vi "Autonomous Independent.vi"() -> ()   [LabVIEW 2020]
doc: "This VI is called when autonomous begins, and will automatically be terminated when autonomous ends. You can carry out timed or sensor driven robot movement independently without needing to return to the caller."
uses:
  <vilib>/Rock Robotics/WPI/ThirdParty/REV Robotics/REVLib/Typedef/Spark MAX Control Type.ctl
  <vilib>/Rock Robotics/WPI/Utilities/WPI_GetSetVariantRefNum.vi
  <vilib>/Rock Robotics/Network Tables/NT Read String.vi
  <vilib>/Rock Robotics/Network Tables/NT Write Numeric Array.vi
panel:
  in  "Array of robot movements 2":T1(array[cluster])=[{"X Joystick Value"=0.39393939393939403, "Y Joystick Value"=0.0, "Delay (sec)"=1.0, "Movement Name"="turn"}, {"X Joystick Value"=-0.3737373737373737, "Y Joystick Value"=0.0, "Delay (sec)"=1.0, "Movement Name"="turn back"}] {"Y Joystick Value" scale=1.0..-1.0; "X Joystick Value" scale=-1.0..1.0}
  # "Be sure to right-click and choose Data Operations>>Make Current Value default if you want to save the array values with the VI"
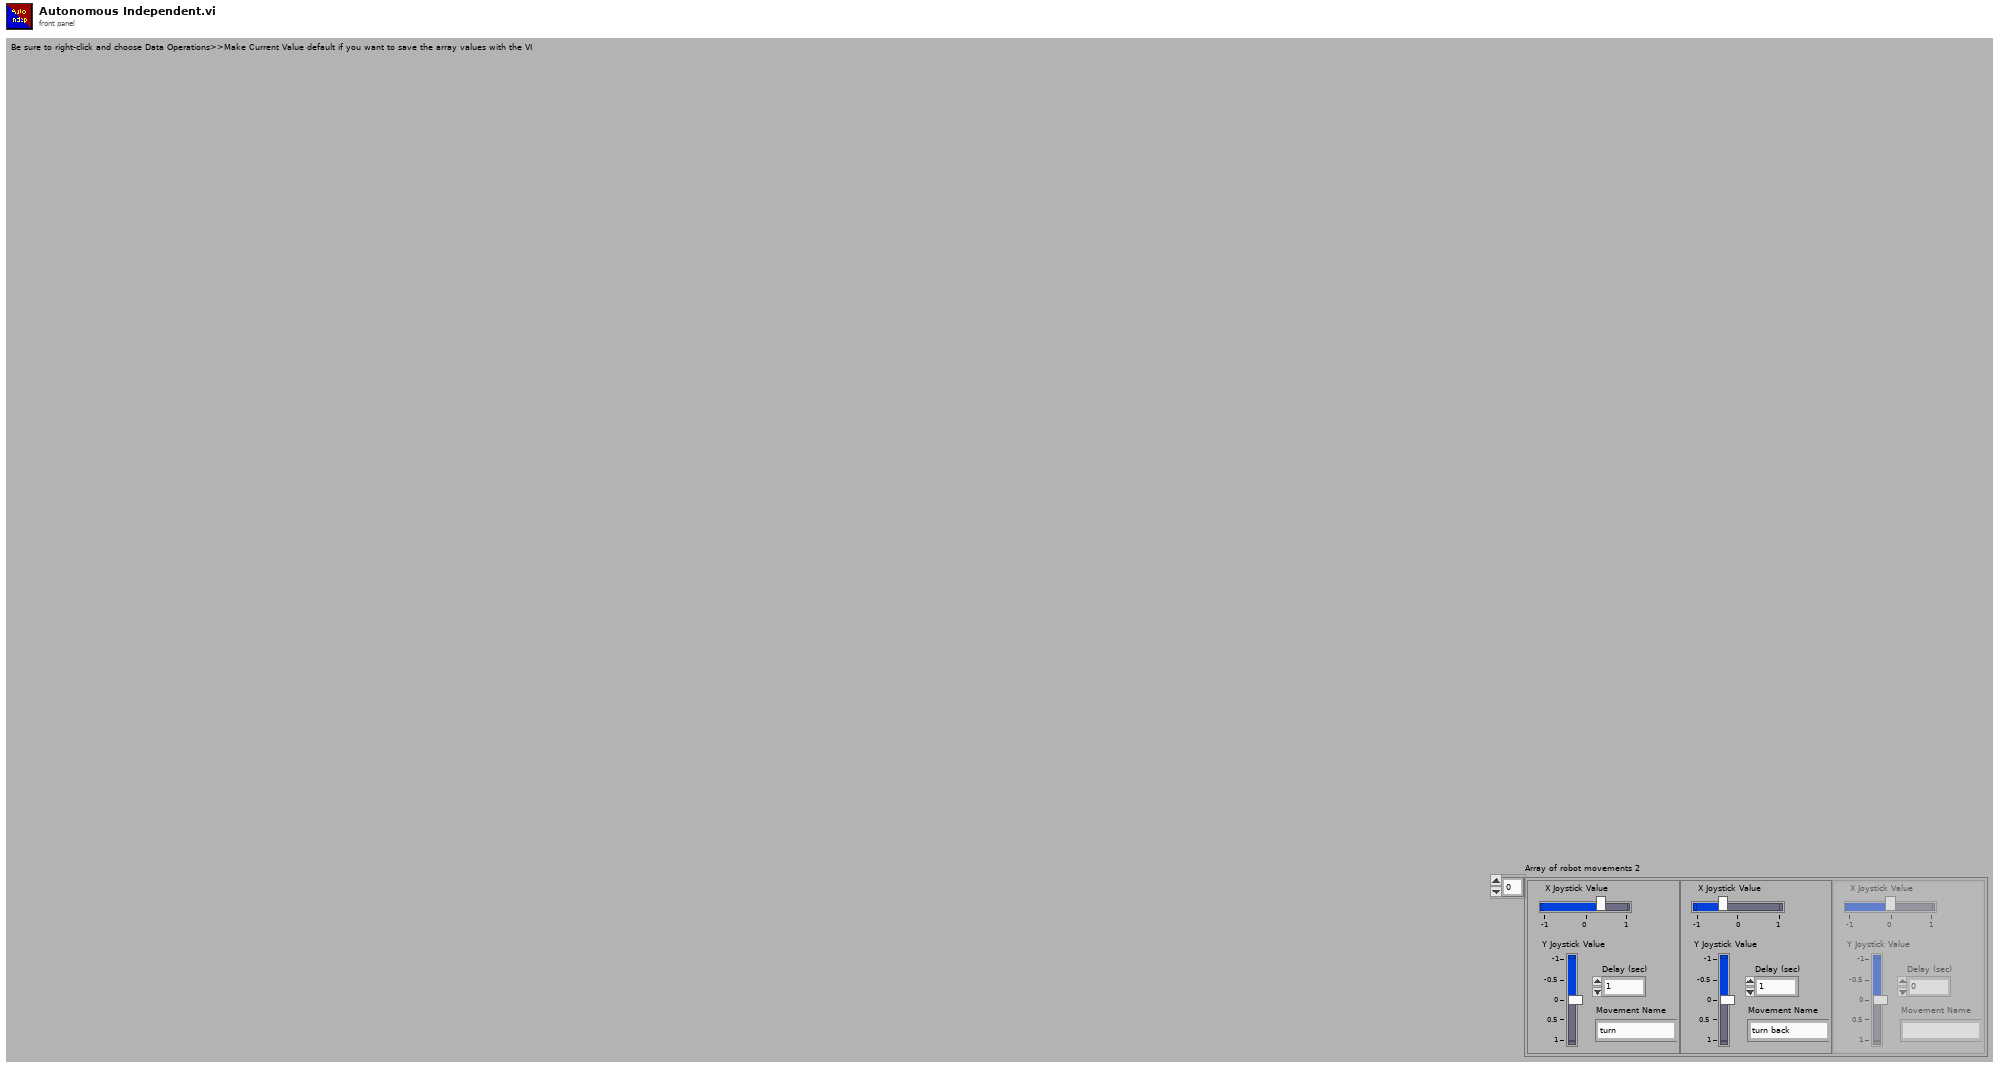
[diagram p1: front panel]
types:
  T1 = cluster{"X Joystick Value":dbl, "Y Joystick Value":dbl, "Delay (sec)":dbl, "Movement Name":string}[]
  T2 = typedef "WPI_JoystickDevRef.ctl" = cluster{"Device":T3}
  T3 = typedef "WPI_JoystickDeviceEnum.ctl" = enum16{"USB 0", "USB 1", "USB 2", "USB 3", "USB 4", "USB 5"}
  T4 = typedef "Spark MAX Control Type.ctl" = enum16{"Percent VBus", "Voltage", "Velocity", "Position", "Smart Motion", "Current", "Smart Velocity"}
  T5 = typedef "WPI_MotorControlDeviceRef.ctl" = cluster{"DeviceStatus":errorcluster, "Type":T6, "PWM":cluster{"PWM Channel":T7, "DeadBand":T8}, "CAN":cluster{"Device Number":u8, "SetOutput VI Ref":variant, "GetOutput VI Ref":variant, "Enable VI Ref":variant, "Disable VI Ref":variant, "Data":variant}, "Invert":bool, "DIO PWM":cluster{"PWM \"Enable\" Channel":T7, "DIOChannel":T9, "PWM Rate":dbl}}
  T6 = typedef "WPI_MotorControlType.ctl" = enum16{"PWM", "CAN", "DIO PWM"}
  T7 = typedef "FPGA_DIOPWMChannel.ctl" = enum8{"PWM 0", "PWM 1", "PWM 2", "PWM 3", "PWM 4", "PWM 5", "PWM 6", "PWM 7", "PWM 8", "PWM 9", "PWM MXP 0", "PWM MXP 1", "PWM MXP 2", "PWM MXP 3", "PWM MXP 4", "PWM MXP 5", "PWM MXP 6", "PWM MXP 7", "PWM MXP 8", "PWM MXP 9", "Invalid"}
  T8 = typedef "WPI_PWMDeadband.ctl" = cluster{"Name":string, "maxPositivePwm":i32, "minPositivePwm":i32, "centerPwm":i32, "maxNegativePwm":i32, "minNegativePwm":i32, "angularRange":u16}
  T9 = typedef "FPGA_DIOChannel.ctl" = enum8{"DIO 0", "DIO 1", "DIO 2", "DIO 3", "DIO 4", "DIO 5", "DIO 6", "DIO 7", "DIO 8", "DIO 9", "DIO MXP 0", "DIO MXP 1", "DIO MXP 2", "DIO MXP 3", "DIO MXP 4", "DIO MXP 5", "DIO MXP 6", "DIO MXP 7", "DIO MXP 8", "DIO MXP 9", "DIO MXP 10", "DIO MXP 11", "DIO MXP 12", "DIO MXP 13", "DIO MXP 14", "DIO MXP 15", "SPI Port CS1", "SPI Port CS2", "SPI Port CS3", "SPI Port MISO", "SPI Port MOSI", "Invalid"}
  T10 = typedef "WPI_RobotDriveDevRef.ctl" = cluster{"DevStatus":errorcluster, "Motors[]":T5[], "Square Inputs":bool, "Max Output":dbl}
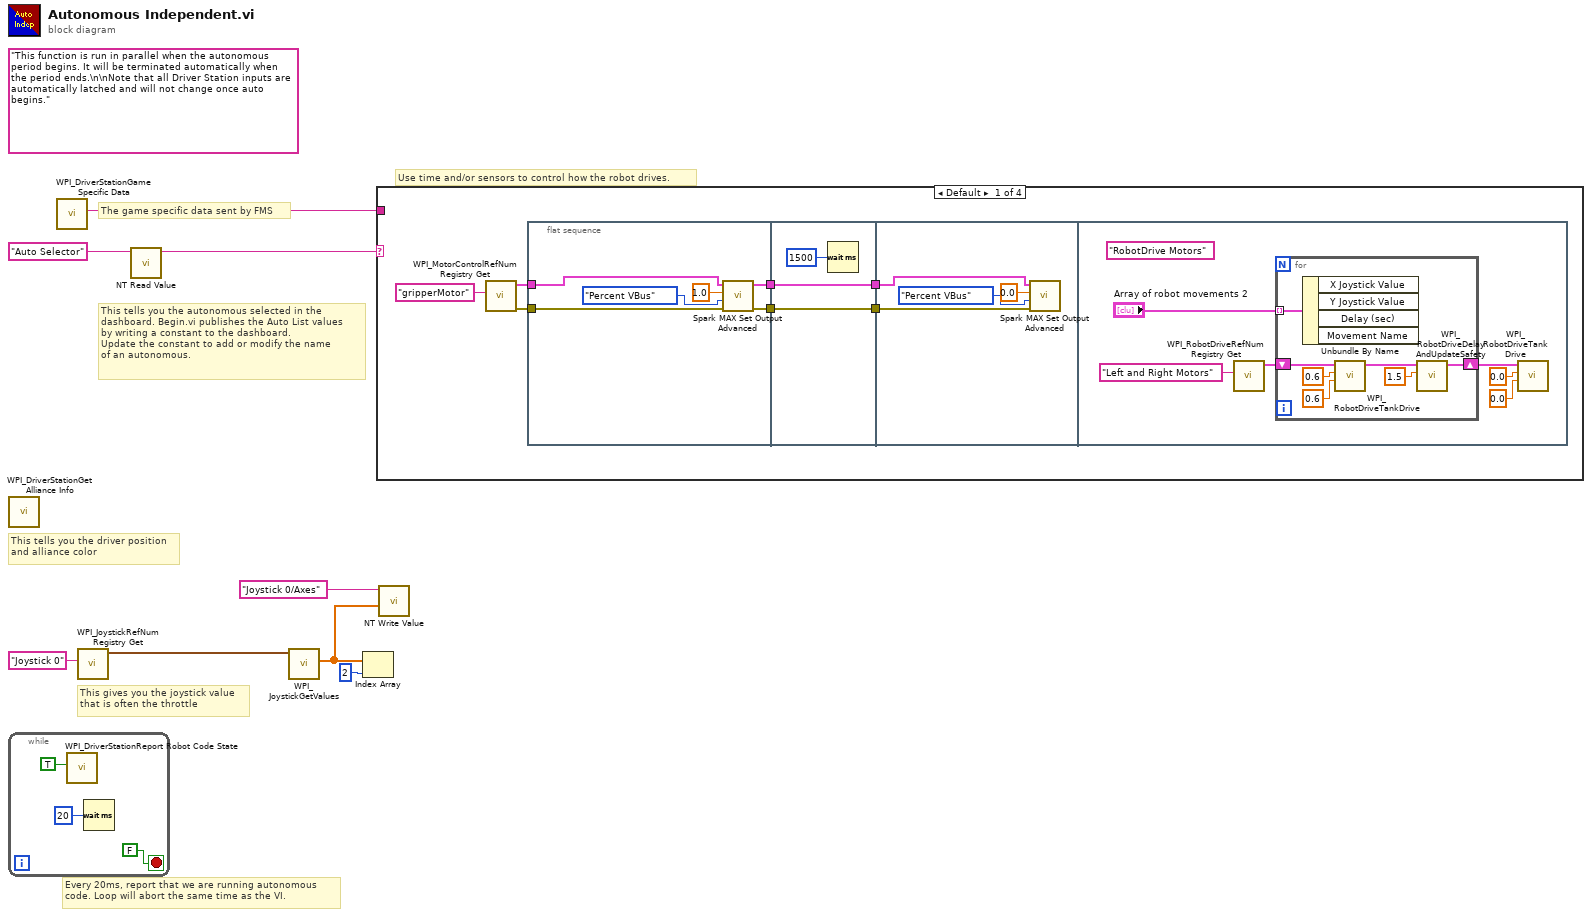
[diagram p0: block diagram]
diagram:
  (unwired) "This function is run in parallel when the autonomous period begins. It will be terminated automatically when the period ends.\n\nNote that all Driver Station inputs are automatically latched and will not change once auto begins."
  # "The game specific data sent by FMS"
  # "This tells you the autonomous selected in the \ndashboard. Begin.vi publishes the Auto List values\nby writing a constant to the dashboard.\nUpdate the constant to add or modify the name\nof an autonomous."
  # "Every 20ms, report that we are running autonomous\ncode. Loop will abort the same time as the VI."
  # "This gives you the joystick value\nthat is often the throttle"
  # "Use time and/or sensors to control how the robot drives."
  # "This tells you the driver position\nand alliance color"
  n1 = call <vilib>:"WPI_DriverStationGet Alliance Info.vi"() -> ()  [unwired: 12 out]
  n2 = while {
    stop <- FALSE stop-if-true
    n3 = call <vilib>:"WPI_DriverStationReport Robot Code State.vi"("Autonomous"=TRUE) -> ()  [unwired: 10 in, 1 out]
    n4 = Wait (ms)(milliseconds to wait=u32 20) -> ()  [unwired: 1 out]
  }
  n5 = call <vilib>:"WPI_DriverStationGame Specific Data.vi"() -> ("Game Specific Data"=w1:string)  [unwired: 11 in]
  n6 = call <vilib>:"WPI_JoystickRefNum Registry Get.vi"("refnum name"="Joystick 0") -> ("JoystickDevRef"=w7:T2)  [unwired: 1 in, 9 out]
  n7 = call-poly <vilib>:"NT Read Value.vi"("name"="Auto Selector" ("Name")) -> ("value"=w4:string)  [unwired: 8 in, 2 out]
  n8 = call <vilib>:"WPI_JoystickGetValues.vi"("JoystickDevRef"=w7) -> ("Axes"=w3:dbl[])  [unwired: 6 in, 4 out]
  n9 = Index Array(array=w3, index=2) -> ()  [unwired: 1 out]
  n10 = case shown="Default" w4 {
    tunnel: w1 -> [_ _ _ _]
    frame Default {
      n11 = call <vilib>:"WPI_MotorControlRefNum Registry Get.vi"("refnum name"="gripperMotor") -> ("error out"=w16:errorcluster, "MotorControlDevRef"=w17:T5)  [unwired: 9 in]
      n12 = flat-sequence {
        tunnel: w17 -> [w24]
        tunnel: w16 -> [w23]
        tunnel: [w20] -> w15
        tunnel: [w19] -> w12
        tunnel: w15 -> [w26]
        tunnel: [w26] -> w14
        tunnel: [w25] -> w13
        tunnel: w12 -> [w25]
        tunnel: w14 -> [w29]
        tunnel: w13 -> [w28]
        frame #0 {
          n13 = call <vilib>:"Spark MAX Set Output Advanced.vi"("error in (no error)"=w23, "Control Mode"=Spark_MAX_Control_Type."Percent VBus", "Setpoint"=1.0, "MotorControlDevRef"=w24) -> ("error out"=w19:errorcluster, "MotorControlDevRef"=w20:T5)  [unwired: 6 in]
        }
        frame #1 {
          n14 = Wait (ms)(milliseconds to wait=u32 1500) -> ()  [unwired: 1 out]
        }
        frame #2 {
          n15 = call <vilib>:"Spark MAX Set Output Advanced.vi"("error in (no error)"=w28, "Control Mode"=Spark_MAX_Control_Type."Percent VBus", "Setpoint"=0.0, "MotorControlDevRef"=w29) -> ()  [unwired: 6 in, 2 out]
        }
        frame #3 {
          (unwired) "RobotDrive Motors" ("Name")
          n16 = call <vilib>:"WPI_RobotDriveRefNum Registry Get.vi"("refnum name"="Left and Right Motors") -> ("RobotDriveDevRef"=w36:T10)  [unwired: 1 in, 9 out]
          n17 = for {
            shift-right: [w44] -> w34
            shift-left: w36 -> [w41]
            tunnel: "Array of robot movements 2" -> [w43] mode=indexing
            n18 = Unbundle By Name(w43) -> ()  [unwired: 4 out]
            n19 = call <vilib>:"WPI_RobotDriveTankDrive.vi"("Right axis value"=0.6 ("Y axis value"), "Left axis value"=0.6 ("X axis value"), "RobotDriveDevRef"=w41) -> ("RobotDriveDevRef"=w38:T10)  [unwired: 6 in, 2 out]
            n20 = call <vilib>:"WPI_RobotDriveDelayAndUpdateSafety.vi"("Delay (s)"=1.5, "RobotDriveDevRef"=w38) -> ("RobotDriveDevRef 2"=w44:T10)  [unwired: 8 in, 1 out]
          }
          n21 = call <vilib>:"WPI_RobotDriveTankDrive.vi"("Right axis value"=0.0 ("X axis value"), "Left axis value"=0.0 ("X axis value"), "RobotDriveDevRef"=w34) -> ()  [unwired: 6 in, 3 out]
        }
      }
    }
    frame "Alternative 1" {
    }
    frame "Alternative 2" {
    }
    frame "Your Turn" {
    }
  }
  n22 = call-poly <vilib>:"NT Write Value.vi"("value"=w3, "name"="Joystick 0/Axes" ("Name")) -> ()  [unwired: 9 in, 1 out]
